vi "条件结构.vi"() -> ()   [LabVIEW 2023]
panel:
  in  "o":dbl
  in  "w":dbl
  in  "y":dbl
  in  "x":dbl
  in  "b":dbl
  in  "a":dbl
  out "Array 7":i32[](array[numeric])
  out "Array 6":i32[](array[numeric])
  out "Array 5":i32[](array[numeric])
  out "Array 4":bool[](array[boolean])
  out "Array 3":bool[](array[boolean])
  out "Array 2":bool[](array[boolean])
  out "Array":bool[](array[boolean])
  in  "example 3":dbl
  in  "example 2":string
  in  "example 1":dbl
  # "条件结构"
  # "1. 注意每个值输入，都要有条件对应，而且， 每个值输入，都要有唯一的条件满足。 不可能一个输入满足多个条件，或者一个条件也不满足。 所以设定  Defalut 是必要的"
  # "尤其值得一提的是，当条件是一个 枚举类型 的时候，它的值的个数是有限的，我们可以在条件结构中为每个条件都设置好相应的分支。\n但是，将来程序可能会出现变动，可能会在枚举类型中添加一个新的条目，或改动某个条目的名字。如果条件结构没有默认分支，作为条件的枚举类型一旦改动，VI 就会出错；\n而如果条件结构有默认分支，则 VI 不会报错，还能运行。"
  # "还是以枚举类型条件为例，程序最开始设计条件结构时，很可能并没有预料到将来会添加一个条件值。这个新添加的条件值，有可能是需要在条件结构中做一些特殊处理的。如果 VI 在改动枚举类型后，\n并不报错，程序员就有可能忘记去更新条件结构，这就是个隐患。相反，如果条件结构中没有默认分支，枚举类型被改动后，VI 会报错，就相当于强迫程序员必须去更新条件结构。\n这可能是一个比较违反最初直觉的原则：如果程序有可能出错，那么我们会希望它越早出错越好，错误越严重越好，最好能够在编译时就报错。"
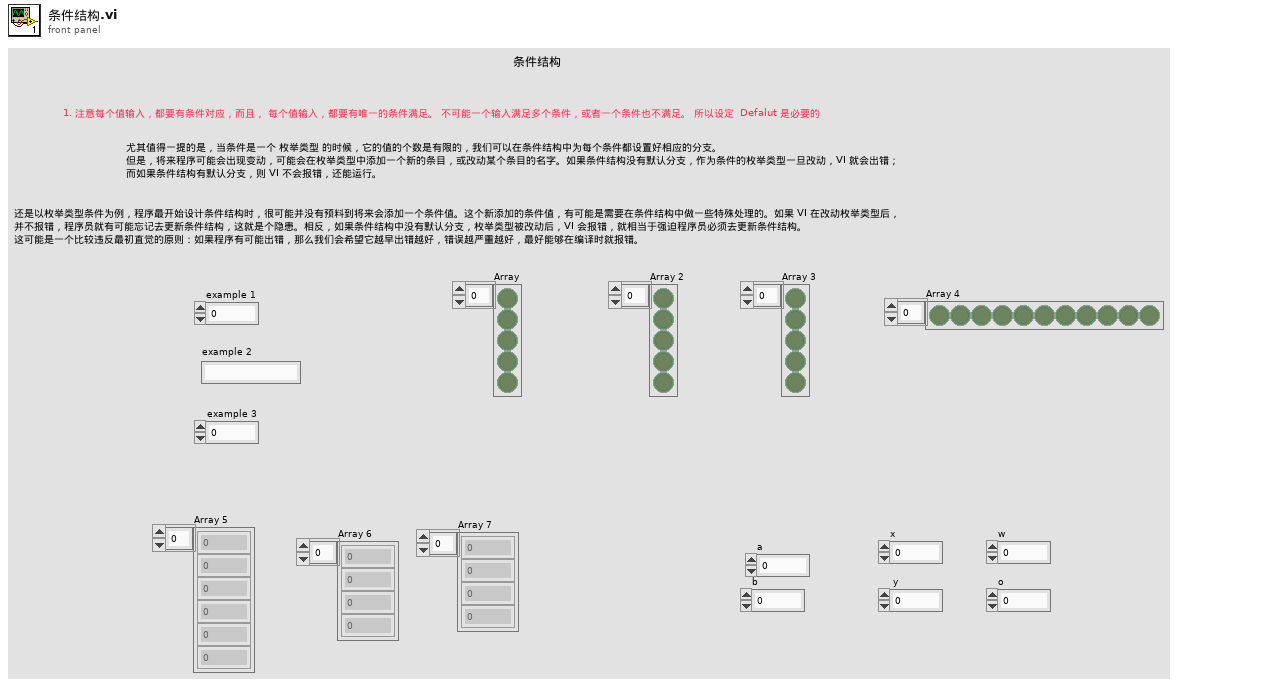
[diagram p1: front panel]
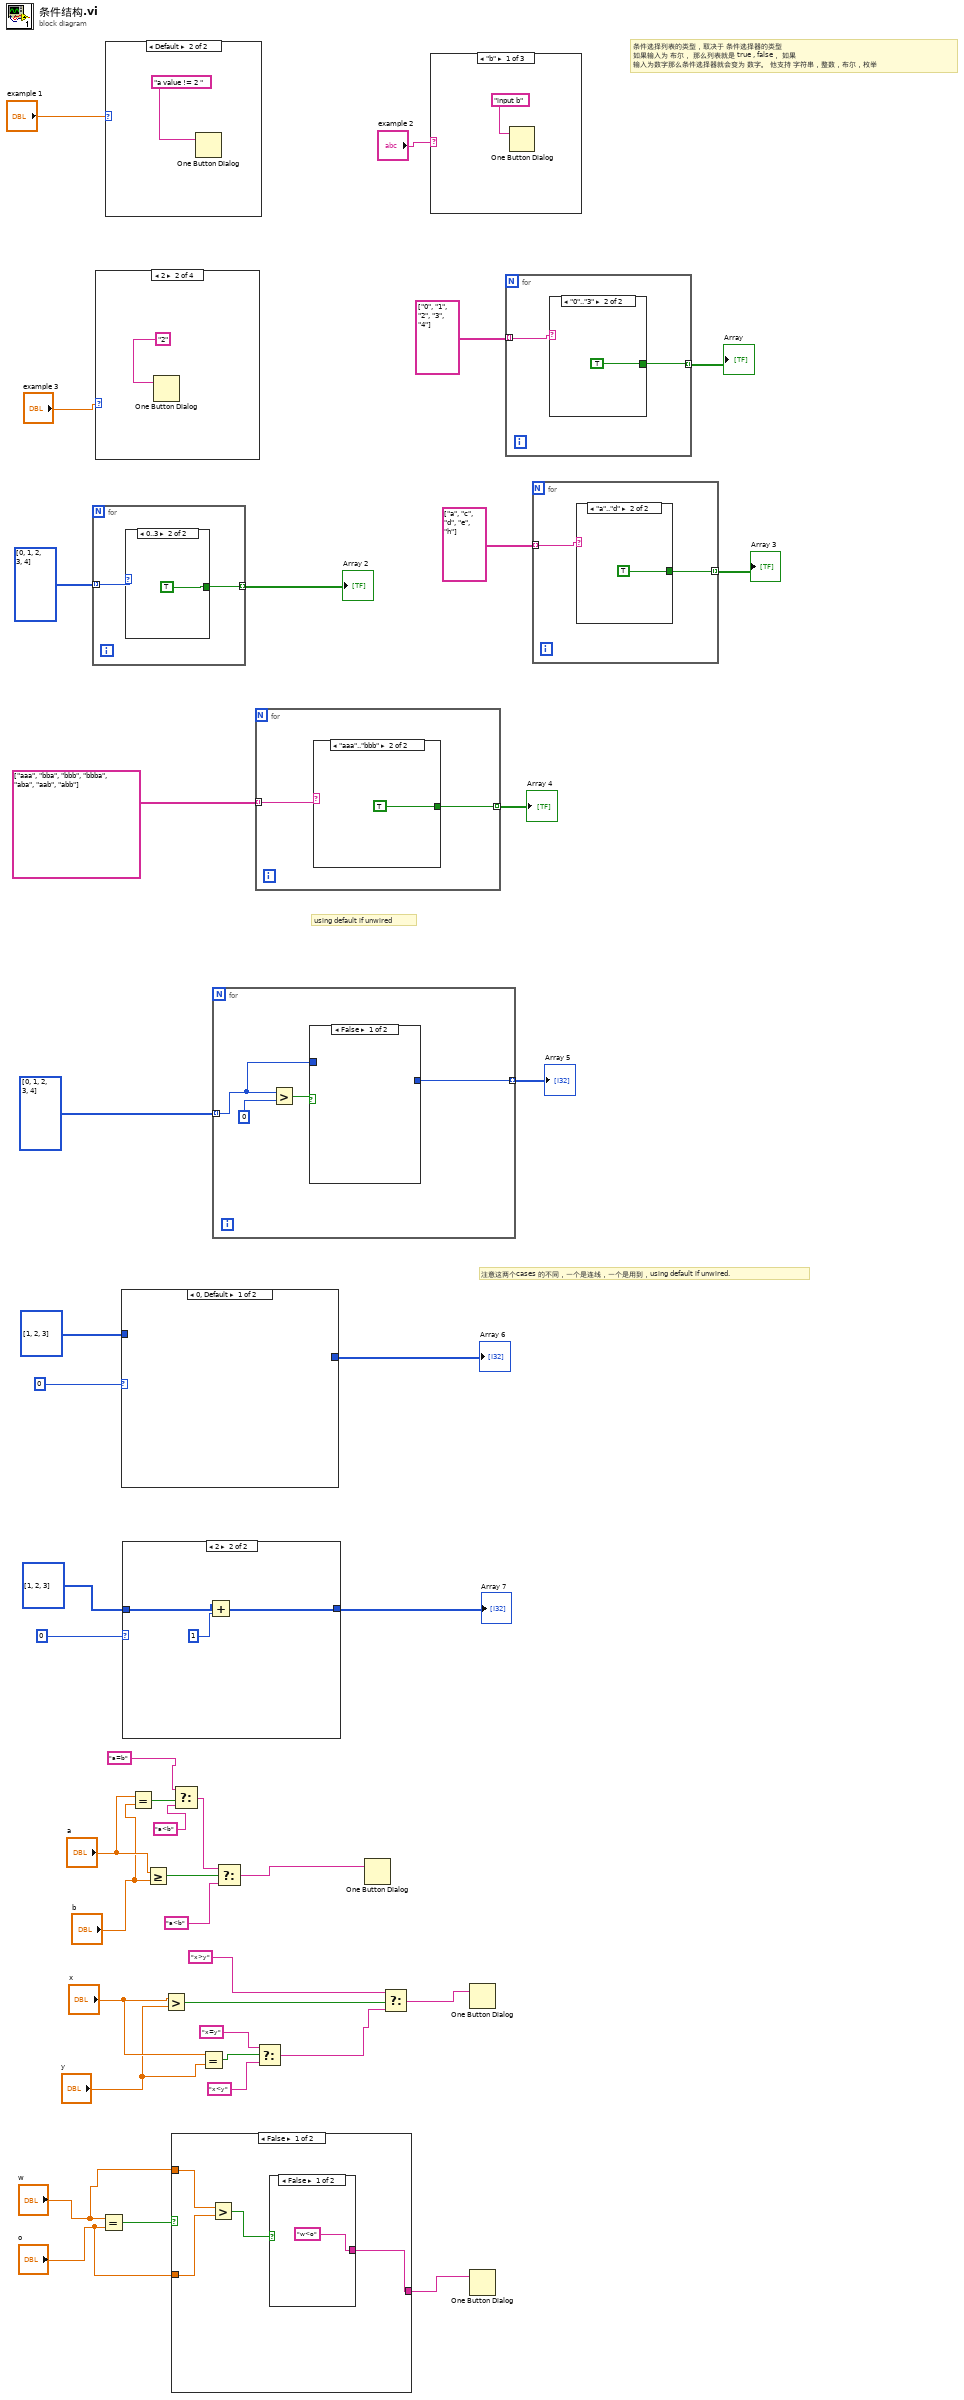
[diagram p0: block diagram]
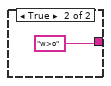
[diagram p2: hidden frame]
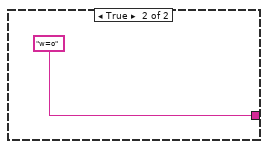
[diagram p3: hidden frame]
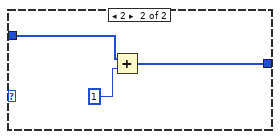
[diagram p5: hidden frame]
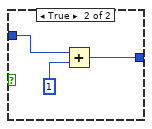
[diagram p6: hidden frame]
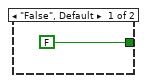
[diagram p7: hidden frame]
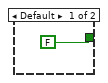
[diagram p8: hidden frame]
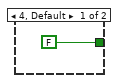
[diagram p9: hidden frame]
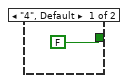
[diagram p10: hidden frame]
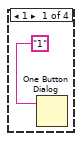
[diagram p11: hidden frame]
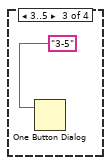
[diagram p12: hidden frame]
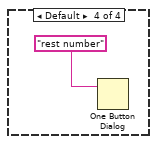
[diagram p13: hidden frame]
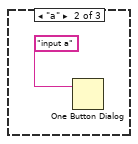
[diagram p14: hidden frame]
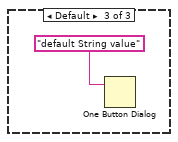
[diagram p15: hidden frame]
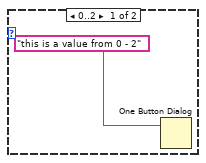
[diagram p16: hidden frame]
diagram:
  # "注意这两个cases 的不同，一个是连线，一个是用到，using default if unwired."
  # "using default if unwired"
  # "条件选择列表的类型，取决于 条件选择器的类型\n如果输入为 布尔， 那么列表就是 true , false， 如果\n输入为数字那么条件选择器就会变为 数字。 他支持 字符串，整数，布尔，枚举"
  n1 = for {
    tunnel: i32[] [0, 1, 2, 3, 4] -> [w43] mode=indexing
    tunnel: [w42] -> w35 mode=indexing
    n2 = case shown="0..3" w43 {
      tunnel: [FALSE TRUE] -> w42
      frame 4, Default {
      }
      frame 0..3 {
      }
    }
  }
  "Array 2" <- w35
  n3 = case shown="2" "example 3" {
    frame 1 {
      n4 = One Button Dialog(message="1") -> ()  [unwired: 1 in, 1 out]
    }
    frame 2 {
      n5 = One Button Dialog(message="2") -> ()  [unwired: 1 in, 1 out]
    }
    frame 3..5 {
      n6 = One Button Dialog(message="3-5") -> ()  [unwired: 1 in, 1 out]
    }
    frame Default {
      n7 = One Button Dialog(message="rest number") -> ()  [unwired: 1 in, 1 out]
    }
  }
  n8 = Equal?(x="w", y="o") -> (x = y?=w4:bool)
  n9 = case shown="Default" "example 1" {
    frame 0..2 {
      n10 = One Button Dialog(message="this is a value from 0 - 2") -> ()  [unwired: 1 in, 1 out]
    }
    frame Default {
      n11 = One Button Dialog(message="a value != 2 ") -> ()  [unwired: 1 in, 1 out]
    }
  }
  n12 = case shown="0, Default" 0 {
    tunnel: i32[] [1, 2, 3] -> [_ w54]
    tunnel: [_ w52] -> w26
    frame 0, Default {
    }
    frame 2 {
      n13 = Add(x=w54, y=1) -> (x+y=w52:i32[])
    }
  }
  "Array 6" <- w26
  n14 = case shown="2" 0 {
    tunnel: i32[] [1, 2, 3] -> [w55 w58]
    tunnel: [w55 w56] -> w23
    frame 0, Default {
    }
    frame 2 {
      n15 = Add(x=w58, y=1) -> (x+y=w56:i32[])
    }
  }
  "Array 7" <- w23
  n16 = Equal?(x="a", y="b") -> (x = y?=w19:bool)
  n17 = Greater Or Equal?(x="a", y="b") -> (x >= y?=w22:bool)
  n18 = Greater?(x="x", y="y") -> (0:w13:bool)
  n19 = case shown="False" w4 {
    tunnel: [w59 "w=o"] -> w3
    tunnel: "w" -> [w62 _]
    tunnel: "o" -> [w61 _]
    frame False {
      n20 = Greater?(x=w62, y=w61) -> (0:w60:bool)
      n21 = case shown="False" w60 {
        tunnel: ["w<o" "w>o"] -> w59
        frame False {
        }
        frame True {
        }
      }
    }
    frame True {
    }
  }
  n22 = Select(t="a=b", s=w19, f="a<b") -> (s? t:f=w20:string)
  n23 = Equal?(x="x", y="y") -> (x = y?=w8:bool)
  n24 = for {
    tunnel: i32[] [0, 1, 2, 3, 4] -> [w67] mode=indexing
    tunnel: [w66] -> w29 mode=indexing
    n25 = Greater?(x=w67, y=0) -> (0:w68:bool)
    n26 = case shown="False" w68 {
      tunnel: w67 -> [_ w72]
      tunnel: [_ w70] -> w66
      frame False {
      }
      frame True {
        n27 = Add(x=w72, y=1) -> (x+y=w70:i32)
      }
    }
  }
  "Array 5" <- w29
  n28 = Select(t=w20, s=w22, f="a<b") -> (s? t:f=w14:string)
  n29 = for {
    tunnel: string[] ["aaa", "bba", "bbb", "bbba", "aba", "aab", "abb"] -> [w74] mode=indexing
    tunnel: [w73] -> w31 mode=indexing
    n30 = case shown="\"aaa\"..\"bbb\"" w74 {
      tunnel: [FALSE TRUE] -> w73
      frame "False", Default {
      }
      frame "aaa".."bbb" {
      }
    }
  }
  "Array 4" <- w31
  n31 = Select(t="x=y", s=w8, f="x<y") -> (s? t:f=w9:string)
  n32 = One Button Dialog(message=w14) -> ()  [unwired: 1 in, 1 out]
  n33 = Select(t="x>y", s=w13, f=w9) -> (s? t:f=w5:string)
  n34 = case shown="\"b\"" "example 2" {
    frame "b" {
      n35 = One Button Dialog(message="input b") -> ()  [unwired: 1 in, 1 out]
    }
    frame "a" {
      n36 = One Button Dialog(message="input a") -> ()  [unwired: 1 in, 1 out]
    }
    frame Default {
      n37 = One Button Dialog(message="default String value") -> ()  [unwired: 1 in, 1 out]
    }
  }
  n38 = One Button Dialog(message=w5) -> ()  [unwired: 1 in, 1 out]
  n39 = One Button Dialog(message=w3) -> ()  [unwired: 1 in, 1 out]
  n40 = for {
    tunnel: string[] ["0", "1", "2", "3", "4"] -> [w81] mode=indexing
    tunnel: [w80] -> w37 mode=indexing
    n41 = case shown="\"0\"..\"3\"" w81 {
      tunnel: [FALSE TRUE] -> w80
      frame "4", Default {
      }
      frame "0".."3" {
      }
    }
  }
  "Array" <- w37
  n42 = for {
    tunnel: string[] ["a", "c", "d", "e", "h"] -> [w85] mode=indexing
    tunnel: [w84] -> w33 mode=indexing
    n43 = case shown="\"a\"..\"d\"" w85 {
      tunnel: [FALSE TRUE] -> w84
      frame Default {
      }
      frame "a".."d" {
      }
    }
  }
  "Array 3" <- w33
